vi "IMU STATUS.vi"(8 "error in (no error)":errorcluster, 11 "YRPHfH":T1) -> (0 "error out":errorcluster, 2 "MAGNETIC Zero for Blue Alliance (deg)":dbl=200.5 format="%#.4f")   [LabVIEW 2023]
uses:
  <vilib>/Analysis/coordinate.llb/Angle Units.ctl
  <vilib>/Analysis/coordinate.llb/Angle Range (Degree).ctl
  <vilib>/Analysis/coordinate.llb/Wrap Angle (scalar).vi
  Global odometry.vi
  <vilib>/Rock Robotics/Network Tables/NT Write Number.vi
  <vilib>/Analysis/NI_AAL_Angle.lvlib
panel:
  in  "string 7":string="MAG/BLUE" caption="magnetic BLUE hdg"
  in  "string 6":string="MAG/delta" caption="delta to mag blue"
  in  "string 5":string="Pitch" caption="Pitch"
  in  "string 4":string="Roll" caption="Roll"
  in  "string 3":string="Yaw" caption="Yaw"
  in  "string 2":string="FHDG" caption="fused heading"
  in  "string":string="HDG" caption="Heading"
  in  "String":string="IMU/" caption="IMU stack"
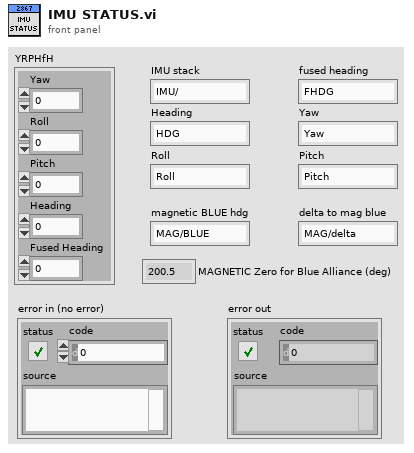
[diagram p1: front panel]
types:
  T1 = cluster{"Yaw":dbl, "Roll":dbl, "Pitch":dbl, "Heading":dbl, "Fused Heading":dbl}
  T2 = typedef "NI_AAL_Angle.lvlib/Angle Range (Degree).ctl" = u16
  T3 = typedef "NI_AAL_Angle.lvlib/Angle Units.ctl" = i32
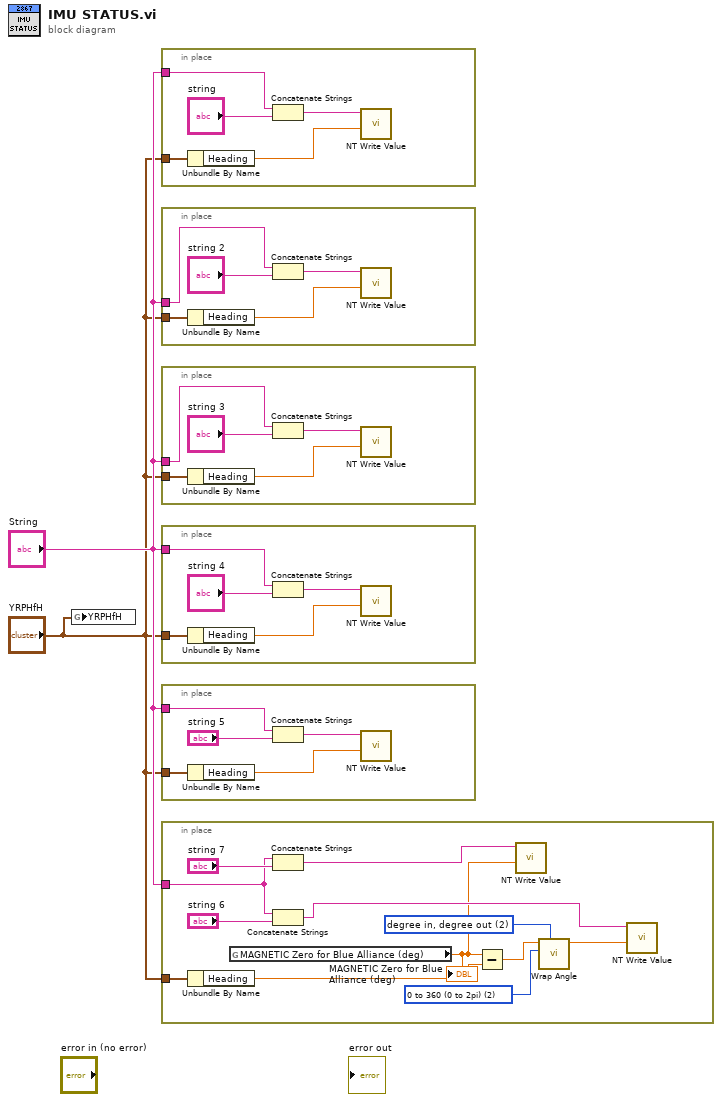
[diagram p0: block diagram]
diagram:
  n1 = global write "Global odometry.vi" "YRPHfH"("YRPHfH") -> ()
  n2 = in-place {
    in-place-border: "YRPHfH" -> [w6]
    in-place-border: "String" -> [w3]
    n3 = Unbundle By Name(w6) -> ("Heading"=w7:dbl)
    n4 = Concatenate Strings(w3, "string") -> (w4:string)
    n5 = call-poly <vilib>:"NT Write Value.vi"("value"=w7, "name"=w4) -> ()  [unwired: 9 in, 1 out]
  }
  n6 = in-place {
    in-place-border: "String" -> [w10]
    in-place-border: "YRPHfH" -> [w9]
    n7 = Unbundle By Name(w9) -> ("Heading"=w8:dbl)
    n8 = Concatenate Strings(w10, "string 2") -> (w11:string)
    n9 = call-poly <vilib>:"NT Write Value.vi"("value"=w8, "name"=w11) -> ()  [unwired: 9 in, 1 out]
  }
  n10 = in-place {
    in-place-border: "String" -> [w15]
    in-place-border: "YRPHfH" -> [w14]
    n11 = Unbundle By Name(w14) -> ("Heading"=w13:dbl)
    n12 = Concatenate Strings(w15, "string 3") -> (w16:string)
    n13 = call-poly <vilib>:"NT Write Value.vi"("value"=w13, "name"=w16) -> ()  [unwired: 9 in, 1 out]
  }
  n14 = in-place {
    in-place-border: "String" -> [w20]
    in-place-border: "YRPHfH" -> [w19]
    n15 = Unbundle By Name(w19) -> ("Heading"=w18:dbl)
    n16 = Concatenate Strings(w20, "string 4") -> (w21:string)
    n17 = call-poly <vilib>:"NT Write Value.vi"("value"=w18, "name"=w21) -> ()  [unwired: 9 in, 1 out]
  }
  n18 = in-place {
    in-place-border: "String" -> [w25]
    in-place-border: "YRPHfH" -> [w24]
    n19 = Unbundle By Name(w24) -> ("Heading"=w23:dbl)
    n20 = Concatenate Strings(w25, "string 5") -> (w26:string)
    n21 = call-poly <vilib>:"NT Write Value.vi"("value"=w23, "name"=w26) -> ()  [unwired: 9 in, 1 out]
  }
  n22 = in-place {
    in-place-border: "String" -> [w30]
    in-place-border: "YRPHfH" -> [w37]
    w33 = T2 2 items=["none", "-180 to 180 (-pi to pi)", "0 to 360 (0 to 2pi)"] ("angle range")
    w34 = T3 2 items=["radian in, radian out", "radian in, degree out", "degree in, degree out", "degree in, radian out"] ("angle units")
    n23 = Unbundle By Name(w37) -> ("Heading"=w29:dbl)
    n24 = global read "Global odometry.vi" "MAGNETIC Zero for Blue Alliance (deg)"() -> (w28:dbl)
    "MAGNETIC Zero for Blue Alliance (deg)" <- w28
    n25 = Concatenate Strings(w30, "string 7") -> (w31:string)
    n26 = Concatenate Strings(w30, "string 6") -> (w38:string)
    n27 = Subtract(x=w28, y=w29) -> (x-y=w36:dbl)
    n28 = call-poly <vilib>:"NT Write Value.vi"("value"=w28, "name"=w31) -> ()  [unwired: 9 in, 1 out]
    n29 = call-poly <vilib>:"Wrap Angle.vi"("angle units"=w34, "angle range"=w33, "angle in"=w36) -> ("angle out"=w35:dbl)  [unwired: 7 in, 1 out]
    n30 = call-poly <vilib>:"NT Write Value.vi"("value"=w35, "name"=w38) -> ()  [unwired: 9 in, 1 out]
  }
